vi "SubVi.Sorting an ini file using a array.vi"(4 "Input data":T2(array[cluster]), 7 "Data in the cluster":T1) -> (1 "Output data":T2(array[cluster]))   [LabVIEW 2015]
doc: "Sorting the ini file data using an array"
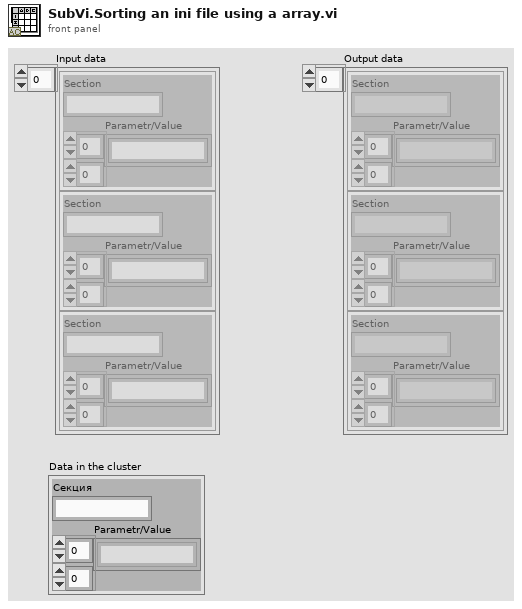
[diagram p1: front panel]
types:
  T1 = cluster{"Секция":string, "Parametr/Value":string[][]}
  T2 = cluster{"Section":string, "Parametr/Value":string[][]}[]
  T3 = cluster{"Секция":string, "Parametr/Value":string[][]}[]
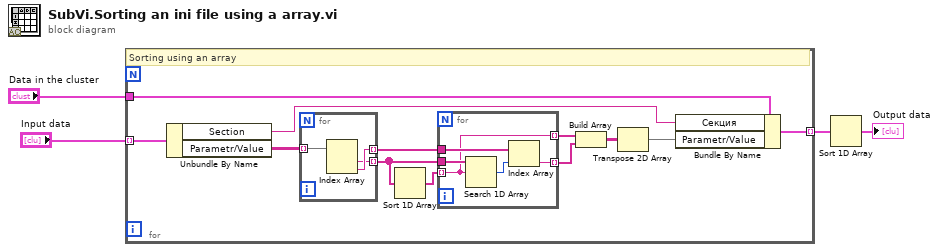
[diagram p0: block diagram]
diagram:
  n1 = for {
    tunnel: "Data in the cluster" -> [w5]
    tunnel: [w16] -> w1 mode=indexing
    tunnel: "Input data" -> [w6] mode=indexing
    # "Sorting using an array"
    n2 = Unbundle By Name(w6) -> ("Section"=w15:string, "Parametr/Value"=w8:string[][])
    n3 = for {
      tunnel: [w19] -> w14 mode=indexing
      tunnel: [w18] -> w12 mode=indexing
      tunnel: w8 -> [w17] mode=indexing
      n4 = Index Array(array=w17) -> (element #1=w18:string, element #2=w19:string)  [unwired: 2 in]
    }
    n5 = Sort 1D Array(array=w12) -> (sorted array=w13:string[])
    n6 = for {
      tunnel: w14 -> [w23]
      tunnel: w13 -> [w20] mode=indexing
      tunnel: w12 -> [w24]
      tunnel: [w21] -> w10 mode=indexing
      tunnel: [w20] -> w9 mode=indexing
      n7 = Search 1D Array(1D array=w24, element=w20) -> (index of element=w22:i32)  [unwired: 1 in]
      n8 = Index Array(array=w23, index=w22) -> (element=w21:string)
    }
    n9 = Build Array(w9, w10) -> (w11:string[][])
    n10 = Transpose 2D Array(2D array=w11) -> (transposed array=w7:string[][])
    n11 = Bundle By Name(cluster=w5, "Секция"=w15, "Parametr/Value"=w7) -> (w16:T1)
  }
  n12 = Sort 1D Array(array=w1) -> (sorted array=→"Output data":T3)
